vi "oax_Cursor Relocate.vi"(8 "error in (no error)":errorcluster, 11 "Order waveform":refnum<vi>) -> (0 "error out":errorcluster)   [LabVIEW 2017]
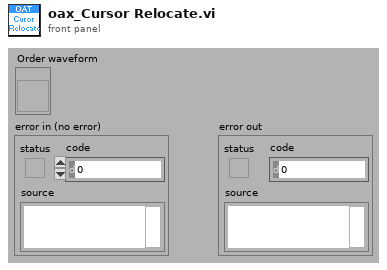
[diagram p1: front panel]
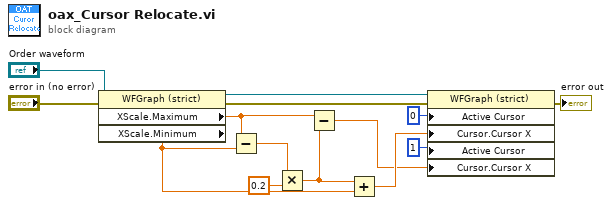
[diagram p0: block diagram]
diagram:
  n1 = property on="Property Node" class="WFGraph (strict)"(reference="Order waveform", error in="error in (no error)") -> (reference out=w5:refnum<vi>, error out=w2:errorcluster, "XScale.Maximum"=w7:dbl, "XScale.Minimum"=w3:dbl)
  n2 = Subtract(x=w7, y=w3) -> (x-y=w10:dbl)
  n3 = Multiply(x=w10, y=0.2) -> (x*y=w4:dbl)
  n4 = Subtract(x=w7, y=w4) -> (x-y=w6:dbl)
  n5 = Add(x=w4, y=w3) -> (x+y=w8:dbl)
  n6 = property on="Property Node" class="WFGraph (strict)"(reference=w5, error in=w2, "Active Cursor"=u32 0, "Cursor.Cursor X"=w8, "Active Cursor"=u32 1, "Cursor.Cursor X"=w6) -> (error out=→"error out":errorcluster)  [unwired: 1 out]
